vi "hydraharp_start_stream.vi"(8 "error in (no error)":errorcluster, 11 "hydraharp in":refnum<class "hydraharp.lvclass">) -> (0 "error out":errorcluster, 3 "hydraharp out":refnum<class "hydraharp.lvclass">)   [LabVIEW 2015, in "hydraharp.lvclass"]
uses:
  hydraharp.lvclass
  hydraharp.lvclass/hydraharp.ctl
  hydraharp_fifo_queue_data.ctl
  hydraharp_fifo_actions.ctl
  hdf5_photon_record_logger/hdf5_photon_record_log.lvclass
  Data Logger Class/data_logger.lvclass
  hhlib.dll
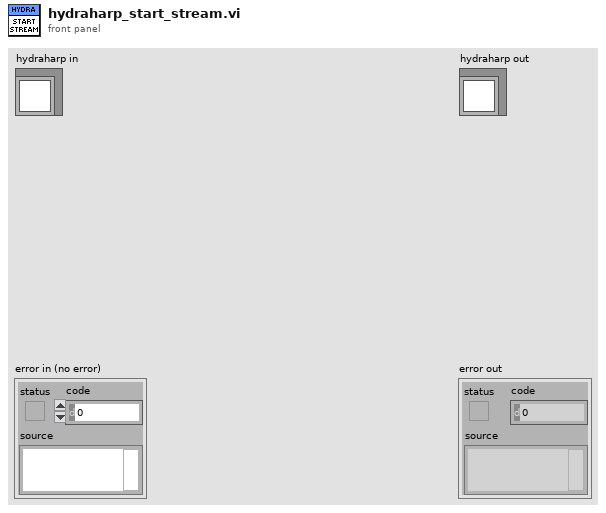
[diagram p1: front panel]
types:
  T1 = typedef "hydraharp_fifo_queue_data.ctl" = cluster{"fifo_buffer":u32[], "fifo_action":T2}
  T2 = typedef "hydraharp_fifo_actions.ctl" = enum16{"stop", "new_data"}
  T3 = typedef "hydraharp_action_on_records.ctl" = enum16{"stream_to_file", "correlate", "stream to file and correlate"}
  T4 = typedef "hpanel_acq_modes.ctl" = u16
  T5 = typedef "record_type.ctl" = enum16{"Raw Stream", "Processed Records (hdf5)"}
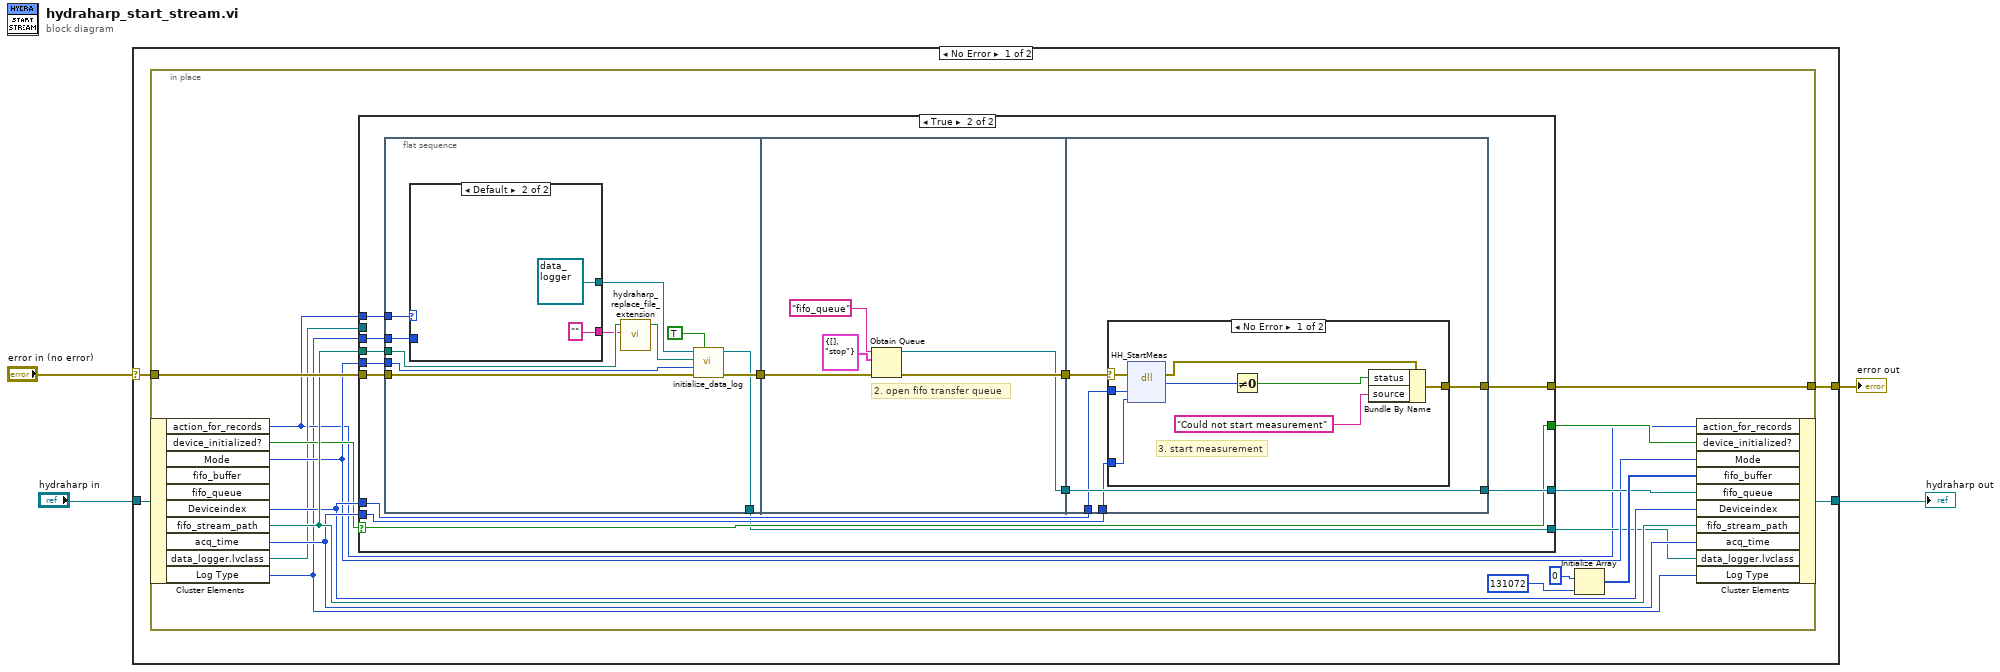
[diagram p0: block diagram]
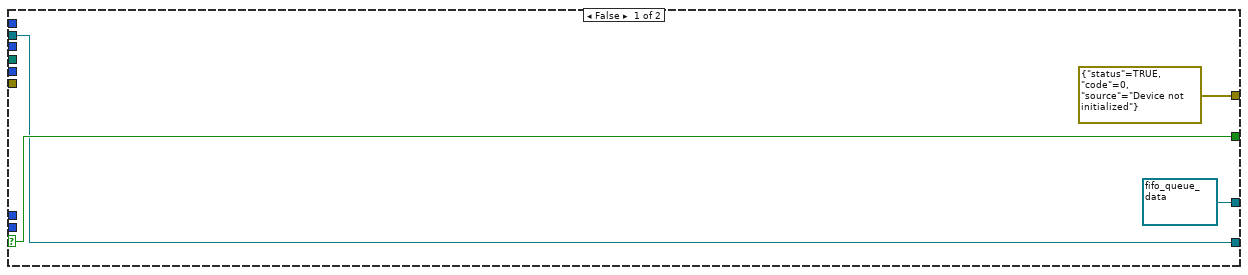
[diagram p2: hidden frame]
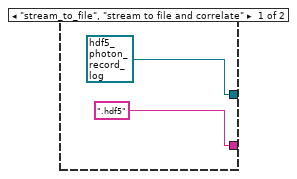
[diagram p3: hidden frame]
diagram:
  n1 = case shown="No Error" "error in (no error)" {
    selector: "error in (no error)" -> [w7 w78]
    tunnel: [w5 w78] -> w3
    tunnel: [w6 w77] -> w1
    tunnel: "hydraharp in" -> [w8 w77]
    frame No Error {
      n2 = in-place {
        in-place-border: w7 -> [w21]
        in-place-border: [w17] -> w5
        n3 = in-place-cluster #1(w8) -> ("action_for_records"=w10:T3, "device_initialized?"=w15:bool, "Mode"=w13:T4, "Deviceindex"=w16:i32, "fifo_stream_path"=w20:path, "acq_time"=w18:i32, "data_logger.lvclass"=w11:refnum<class "data_logger.lvclass">, "Log Type"=w9:T5)  [unwired: 2 out]
        n4 = case shown="True" w15 {
          selector: w15 -> [w26 w33]
          tunnel: w21 -> [_ w40]
          tunnel: w20 -> [_ w39]
          tunnel: [refnum<queue> refnum ("queue out") w38] -> w19
          tunnel: w18 -> [_ w37]
          tunnel: [errorcluster {"status"=TRUE, "code"=0, "source"="Device not initialized"} ("error IO") w36] -> w17
          tunnel: w16 -> [_ w35]
          tunnel: w13 -> [_ w34]
          tunnel: [w26 w33] -> w14
          tunnel: [w25 w31] -> w12
          tunnel: w11 -> [w25 _]
          tunnel: w10 -> [_ w30]
          tunnel: w9 -> [_ w29]
          frame False {
          }
          frame True {
            n5 = flat-sequence {
              tunnel: w40 -> [w50]
              tunnel: w39 -> [w53]
              tunnel: [w51] -> w32
              tunnel: w34 -> [w52]
              tunnel: [w49] -> w31
              tunnel: w30 -> [w45]
              tunnel: w29 -> [w44]
              tunnel: [w59] -> w42
              tunnel: [w58] -> w41
              tunnel: w32 -> [w60]
              tunnel: [w67] -> w38
              tunnel: w42 -> [w63]
              tunnel: w41 -> [w67]
              tunnel: w37 -> [w66]
              tunnel: [w65] -> w36
              tunnel: w35 -> [w64]
              frame #0 {
                n6 = case shown="Default" w45 {
                  tunnel: [refnum<class "hdf5_photon_record_log.lvclass"> refnum ("hdf5_photon_record_log.lvclass") refnum<class "data_logger.lvclass"> refnum ("data_logger.lvclass")] -> w47
                  tunnel: w44 -> [_ _]
                  tunnel: [".hdf5" ("new_extension") "" ("new_extension")] -> w43
                  frame "stream_to_file", "stream to file and correlate" {
                  }
                  frame Default {
                  }
                }
                n7 = call "hydraharp_replace_file_extension.vi"("new_extension"=w43, "input_file"=w53) -> ("new_name"=w46:path)  [unwired: 9 in]
                n8 = call-dynamic "initialize_data_log.vi"("Overwrite?"=TRUE, "error in (no error)"=w50, "Initialization Data"=w52, "Path"=w46, "data_logger in"=w47) -> ("error out"=w51:errorcluster, "data_logger out"=w49:refnum<class "data_logger.lvclass">)  [unwired: 5 in]
              }
              frame #1 {
                # "2. open fifo transfer queue"
                n9 = Obtain Queue(name (unnamed)="fifo_queue", element data type=T1 {"fifo_buffer"=[], "fifo_action"=enum."stop"} ("fifo_queue_data"), error in (no error)=w60) -> (queue out=w58:refnum<queue>, error out=w59:errorcluster)  [unwired: 2 in, 1 out]
              }
              frame #2 {
                n10 = case shown="No Error" w63 {
                  selector: w63 -> [w68 w76]
                  tunnel: w66 -> [w75 _]
                  tunnel: [w70 w76] -> w65
                  tunnel: w64 -> [w69 _]
                  frame No Error {
                    # "3. start measurement"
                    n11 = dll-call lib="hhlib.dll" fn="HH_StartMeas"(error in=w68, "devidx"=w69, "tacq"=w75) -> (error out=w73:errorcluster, w74:i32)  [unwired: 4 in, 1 out]
                    n12 = Not Equal To 0?(x=w74) -> (x != 0?=w72:bool)
                    n13 = Bundle By Name(cluster=w73, "status"=w72, "source"="Could not start measurement") -> (w70:errorcluster)
                  }
                  frame Error {
                  }
                }
              }
            }
          }
        }
        n14 = Initialize Array(u32 0 ("element"), 131072 ("dimension size")) -> (w24:u32[])
        n15 = in-place-cluster #1("action_for_records"=w10, "device_initialized?"=w14, "Mode"=w13, "fifo_buffer"=w24, "fifo_queue"=w19, "Deviceindex"=w16, "fifo_stream_path"=w20, "acq_time"=w18, "data_logger.lvclass"=w12, "Log Type"=w9) -> (w6:refnum<class "hydraharp.lvclass">)
      }
    }
    frame Error {
    }
  }
  "error out" <- w3
  "hydraharp out" <- w1
